vi "Tokenise String.vi"(8 "error in (no error)":errorcluster, 10 "Delimiter":string=",", 11 "String to Parse":string) -> (0 "error out":errorcluster, 1 "Tokens Found":bool, 2 "Token Count":i32, 3 "Tokens":string[](array[string]))   [LabVIEW 2023, in "HAF.lvlib"]
uses:
  HAF.lvlib
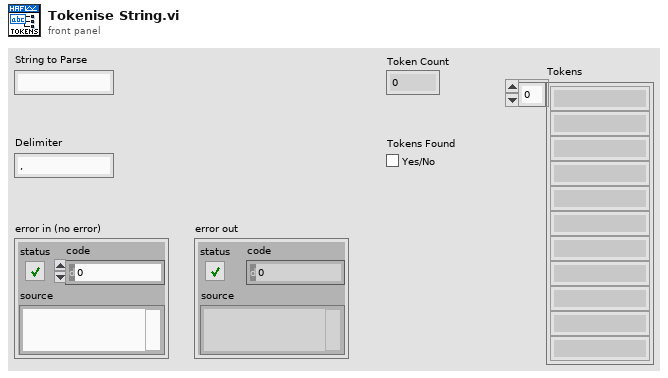
[diagram p1: front panel]
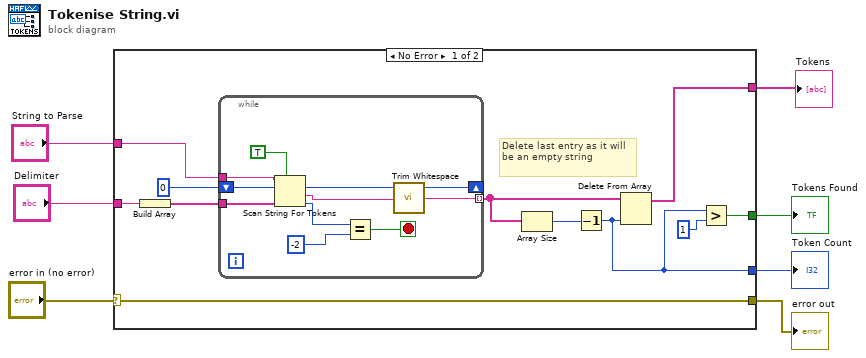
[diagram p0: block diagram]
diagram:
  n1 = case shown="No Error" "error in (no error)" {
    selector: "error in (no error)" -> [w8 w29]
    tunnel: "String to Parse" -> [w18 _]
    tunnel: "Delimiter" -> [w16 _]
    tunnel: [w8 w29] -> w4
    tunnel: [w12 _] -> w3
    tunnel: [w10 _] -> w2
    tunnel: [w9 _] -> w1
    frame No Error {
      # "Delete last entry as it will be an empty string"
      n2 = Build Array(w16) -> (w15:string[])
      n3 = while {
        tunnel: w18 -> [w28]
        tunnel: w15 -> [w26]
        shift-right: [w24] -> _
        shift-left: 0 -> [w27]
        tunnel: [w22] -> w13 mode=indexing
        stop <- w19 stop-if-true
        n4 = Scan String For Tokens(5:TRUE ("allow empty tokens? (F)"), 6:w26, 8:w27, 9:w28) -> (0:w21:i32, 1:w23:string, 2:w24:i32)  [unwired: 2 in, 1 out]
        n5 = Equal?(x=w21, y=-2) -> (x = y?=w19:bool)
        n6 = call <vilib>:"Trim Whitespace.vi"("string"=w23) -> ("trimmed string"=w22:string)  [unwired: 1 in]
      }
      n7 = Array Size(array=w13) -> (size(s)=w14:i32)
      n8 = Decrement(x=w14) -> (x-1=w9:i32)
      n9 = Delete From Array(array=w13, index=w9) -> (array with subset deleted=w12:string[])  [unwired: 1 in, 1 out]
      n10 = Greater?(x=w9, y=1) -> (0:w10:bool)
    }
    frame Error {
    }
  }
  "error out" <- w4
  "Token Count" <- w1
  "Tokens Found" <- w2
  "Tokens" <- w3
